vi "degaus_var_step_size.vi"() -> ()   [LabVIEW 2011]
panel:
  in  "direction":u16(ring)=2 items=["X", "Y", "Z"]
  in  "milliseconds to wait":u32=500
  out "error":bool=TRUE
  in  "max current":dbl=5.0
  out "factor":dbl
  in  "number":i32=50
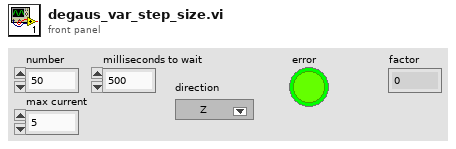
[diagram p1: front panel]
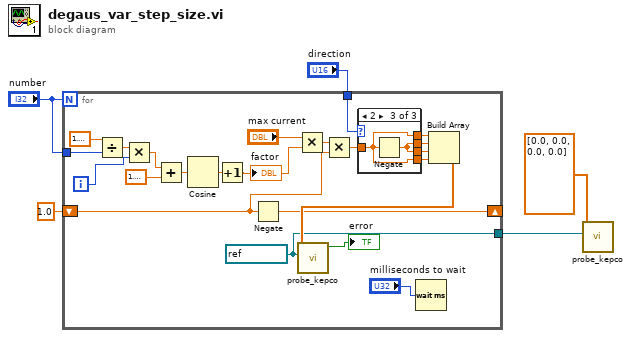
[diagram p0: block diagram]
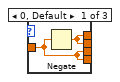
[diagram p2: hidden frame]
diagram:
  n1 = for {
    N: "number" -> [_]
    shift-right: [w24] -> _
    shift-left: 1.0 ("x*y") -> [w25]
    tunnel: "number" -> [w7]
    tunnel: "direction" -> [w22]
    tunnel: [w16] -> w2
    i -> [w8]
    w16 = refnum<visa-resource-name> "COM7" ("VISA-Ressourcenname")
    n2 = Divide(x=1.5707963267948966, y=w7) -> (x/y=w12:dbl)
    n3 = Multiply(x=w12, y=w8) -> (x*y=w11:dbl)
    n4 = Add(x=w11, y=1.5707963267948966) -> (x+y=w10:dbl)
    n5 = Cosine(x=w10) -> (cos(x)=w15:dbl)
    n6 = Increment(x=w15) -> (x+1=w9:dbl)
    "factor" <- w9
    n7 = Negate(x=w25) -> (-x=w24:dbl)
    n8 = Multiply(x="max current", y=w9) -> (x*y=w6:dbl)
    n9 = Multiply(x=w6, y=w25) -> (x*y=w21:dbl)
    n10 = case shown="2" w22 {
      tunnel: w21 -> [w30 w31 w32]
      tunnel: [w29 w31 w32] -> w20
      tunnel: [w29 w31 w33] -> w19
      tunnel: [w30 w31 w33] -> w18
      tunnel: [w30 w31 w32] -> w17
      frame 0, Default {
        n11 = Negate(x=w30) -> (-x=w29:dbl)
      }
      frame 1 {
      }
      frame 2 {
        n12 = Negate(x=w32) -> (-x=w33:dbl)
      }
    }
    n13 = Wait (ms)(milliseconds to wait="milliseconds to wait") -> ()  [unwired: 1 out]
    n14 = Build Array(w20, w19, w18, w17) -> (w26:dbl[])
    n15 = call "probe_kepco.vi"("VISA-Ressourcenname"=w16, "strommatrix"=w26) -> ("Boolesch"=→"error":bool)  [unwired: 9 in]
  }
  n16 = call "probe_kepco.vi"("VISA-Ressourcenname"=w2, "strommatrix"=dbl[] [0.0, 0.0, 0.0, 0.0]) -> ()  [unwired: 9 in, 1 out]
